vi "UpdatePump.vi"(8 "error in (no error)":errorcluster, 9 "DI":refnum<class "Sig_DI_Simple.lvclass">, 10 "DO in":refnum<class "Sig_DO_Simple.lvclass">, 11 "Pump_1AI_1DO_2DI in":refnum<class "Engine_1DI_2DO.lvclass">) -> (0 "error out":errorcluster, 2 "DO out":refnum<class "Sig_DO_Simple.lvclass">, 3 "Pump_1AI_1DO_2DI out":refnum<class "Engine_1DI_2DO.lvclass">)   [LabVIEW 2019, in "Engine_1DI_2DO.lvclass"]
uses:
  Engine_1DI_2DO.lvclass
  Sig_DI_Simple_class/Sig_DI_Simple.lvclass
  Sig_DO_Simple_class/Sig_DO_Simple.lvclass
  D:/H4000/src/Proccess_class/Proccess.lvclass
  Engine_1DI_2DO.lvclass/Engine_1DI_2DO.ctl
  Sig_DI_Simple_class/Sig_DI_Simple.lvclass/Sig_DI_Simple.ctl
  Sig_DA_class/Sig_DA.lvclass/Sig_DA.ctl
  Proccess_class/Proccess.lvclass/Proccess.ctl
  Sig_DO_Simple_class/Sig_DO_Simple.lvclass/Sig_DO_Simple.ctl
  TypeDef/StatePump.ctl
  Sig_DO_Simple_class/private/write_do_to_db.vi
  subvis/bool_change.vi
  Sig_DA_class/private/write_to_db.vi
  Proccess_class/Read TagName.vi
  Proccess_class/Read Logger.vi
  Sig_DA_class/Sig_DA.lvclass
  Logger_class/WriteEvent.vi
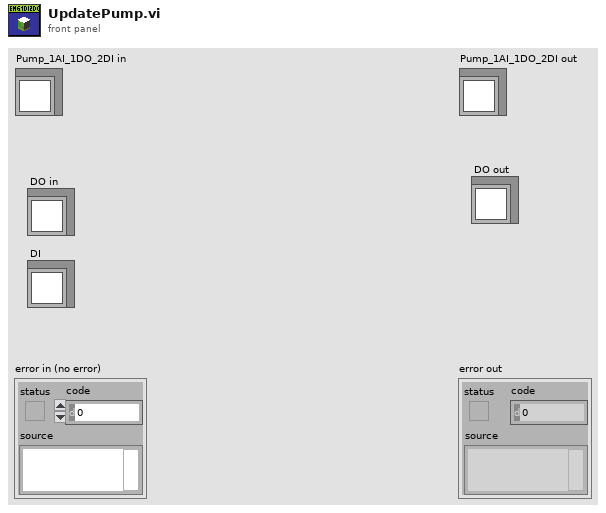
[diagram p1: front panel]
types:
  T1 = typedef "StatePump.ctl" = enum16{"Off", "TupningOn", "On", "TurningOff"}
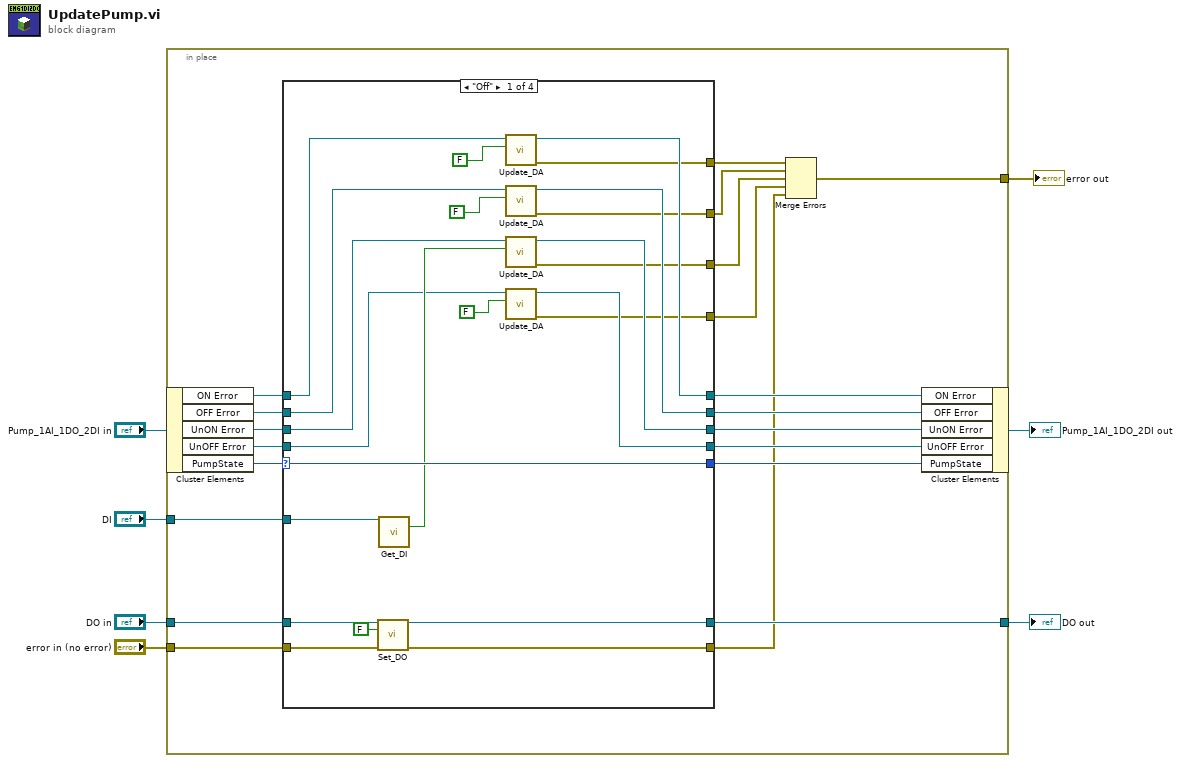
[diagram p0: block diagram]
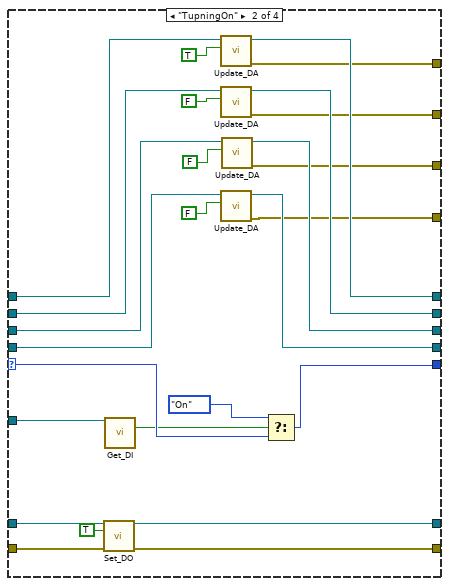
[diagram p2: hidden frame]
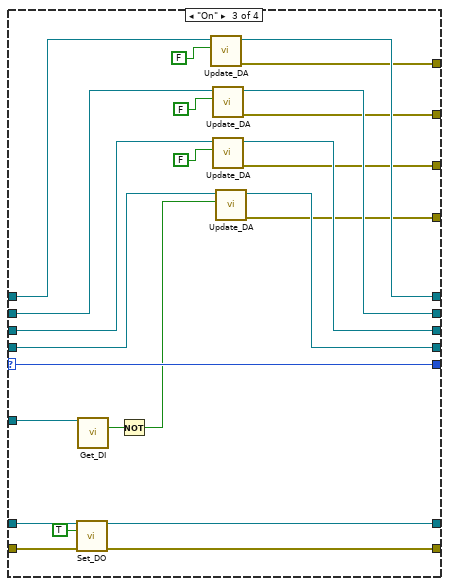
[diagram p3: hidden frame]
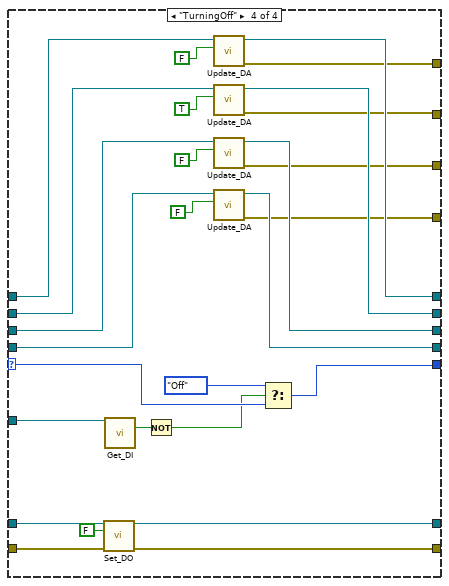
[diagram p4: hidden frame]
diagram:
  n1 = in-place {
    in-place-border: "DI" -> [w26]
    in-place-border: "DO in" -> [w24]
    in-place-border: [w23] -> w1
    in-place-border: "error in (no error)" -> [w22]
    in-place-border: [w8] -> w6
    n2 = in-place-cluster #1("Pump_1AI_1DO_2DI in") -> ("ON Error"=w19:refnum<class "Sig_DA.lvclass">, "OFF Error"=w17:refnum<class "Sig_DA.lvclass">, "UnON Error"=w21:refnum<class "Sig_DA.lvclass">, "UnOFF Error"=w15:refnum<class "Sig_DA.lvclass">, "PumpState"=w27:T1)
    n3 = case shown="\"Off\"" w27 {
      selector: w27 -> [w49 w75 w94 w126]
      tunnel: w26 -> [w50 w76 w100 w127]
      tunnel: [w49 w72 w94 w123] -> w25
      tunnel: w24 -> [w48 w71 w99 w122]
      tunnel: [w47 w70 w98 w121] -> w23
      tunnel: w22 -> [w45 w68 w96 w119]
      tunnel: [w44 w67 w95 w118] -> w9
      tunnel: w21 -> [w43 w58 w86 w108]
      tunnel: [w38 w65 w91 w114] -> w20
      tunnel: w19 -> [w39 w66 w92 w115]
      tunnel: [w35 w59 w87 w111] -> w18
      tunnel: w17 -> [w36 w60 w88 w112]
      tunnel: [w32 w55 w83 w106] -> w16
      tunnel: w15 -> [w33 w56 w84 w107]
      tunnel: [w42 w57 w85 w105] -> w14
      tunnel: [w31 w51 w77 w101] -> w10
      tunnel: [w30 w52 w78 w102] -> w11
      tunnel: [w29 w53 w79 w104] -> w12
      tunnel: [w28 w54 w80 w103] -> w13
      frame "Off" {
        n4 = call "Set_DO.vi"("reference in"=w48, "DO"=FALSE, "error in (no error)"=w45) -> ("reference out"=w47:refnum<class "Sig_DO_Simple.lvclass">, "error out"=w44:errorcluster)  [unwired: 11 in]
        n5 = call "Get_DI.vi"("reference in"=w50) -> ("DI"=w41:bool)  [unwired: 14 in]
        n6 = call "Update_DA.vi"("RAW"=FALSE, "Sig_DA in"=w39) -> ("error out"=w28:errorcluster, "Sig_DA out"=w38:refnum<class "Sig_DA.lvclass">)  [unwired: 7 in, 1 out]
        n7 = call "Update_DA.vi"("RAW"=FALSE, "Sig_DA in"=w36) -> ("error out"=w29:errorcluster, "Sig_DA out"=w35:refnum<class "Sig_DA.lvclass">)  [unwired: 7 in, 1 out]
        n8 = call "Update_DA.vi"("RAW"=w41, "Sig_DA in"=w43) -> ("error out"=w30:errorcluster, "Sig_DA out"=w42:refnum<class "Sig_DA.lvclass">)  [unwired: 7 in, 1 out]
        n9 = call "Update_DA.vi"("RAW"=FALSE, "Sig_DA in"=w33) -> ("error out"=w31:errorcluster, "Sig_DA out"=w32:refnum<class "Sig_DA.lvclass">)  [unwired: 7 in, 1 out]
      }
      frame "TupningOn" {
        n10 = call "Set_DO.vi"("reference in"=w71, "DO"=TRUE, "error in (no error)"=w68) -> ("reference out"=w70:refnum<class "Sig_DO_Simple.lvclass">, "error out"=w67:errorcluster)  [unwired: 11 in]
        n11 = call "Get_DI.vi"("reference in"=w76) -> ("DI"=w74:bool)  [unwired: 14 in]
        n12 = call "Update_DA.vi"("RAW"=TRUE, "Sig_DA in"=w66) -> ("error out"=w54:errorcluster, "Sig_DA out"=w65:refnum<class "Sig_DA.lvclass">)  [unwired: 7 in, 1 out]
        n13 = call "Update_DA.vi"("RAW"=FALSE, "Sig_DA in"=w60) -> ("error out"=w53:errorcluster, "Sig_DA out"=w59:refnum<class "Sig_DA.lvclass">)  [unwired: 7 in, 1 out]
        n14 = call "Update_DA.vi"("RAW"=FALSE, "Sig_DA in"=w56) -> ("error out"=w51:errorcluster, "Sig_DA out"=w55:refnum<class "Sig_DA.lvclass">)  [unwired: 7 in, 1 out]
        n15 = call "Update_DA.vi"("RAW"=FALSE, "Sig_DA in"=w58) -> ("error out"=w52:errorcluster, "Sig_DA out"=w57:refnum<class "Sig_DA.lvclass">)  [unwired: 7 in, 1 out]
        n16 = Select(t=StatePump."On", s=w74, f=w75) -> (s? t:f=w72:T1)
      }
      frame "On" {
        n17 = call "Set_DO.vi"("reference in"=w99, "DO"=TRUE, "error in (no error)"=w96) -> ("reference out"=w98:refnum<class "Sig_DO_Simple.lvclass">, "error out"=w95:errorcluster)  [unwired: 11 in]
        n18 = call "Get_DI.vi"("reference in"=w100) -> ("DI"=w82:bool)  [unwired: 14 in]
        n19 = Not(x=w82) -> (.not. x?=w81:bool)
        n20 = call "Update_DA.vi"("RAW"=FALSE, "Sig_DA in"=w92) -> ("error out"=w80:errorcluster, "Sig_DA out"=w91:refnum<class "Sig_DA.lvclass">)  [unwired: 7 in, 1 out]
        n21 = call "Update_DA.vi"("RAW"=FALSE, "Sig_DA in"=w88) -> ("error out"=w79:errorcluster, "Sig_DA out"=w87:refnum<class "Sig_DA.lvclass">)  [unwired: 7 in, 1 out]
        n22 = call "Update_DA.vi"("RAW"=FALSE, "Sig_DA in"=w86) -> ("error out"=w78:errorcluster, "Sig_DA out"=w85:refnum<class "Sig_DA.lvclass">)  [unwired: 7 in, 1 out]
        n23 = call "Update_DA.vi"("RAW"=w81, "Sig_DA in"=w84) -> ("error out"=w77:errorcluster, "Sig_DA out"=w83:refnum<class "Sig_DA.lvclass">)  [unwired: 7 in, 1 out]
      }
      frame "TurningOff" {
        n24 = call "Set_DO.vi"("reference in"=w122, "DO"=FALSE, "error in (no error)"=w119) -> ("reference out"=w121:refnum<class "Sig_DO_Simple.lvclass">, "error out"=w118:errorcluster)  [unwired: 11 in]
        n25 = call "Get_DI.vi"("reference in"=w127) -> ("DI"=w125:bool)  [unwired: 14 in]
        n26 = Not(x=w125) -> (.not. x?=w117:bool)
        n27 = call "Update_DA.vi"("RAW"=FALSE, "Sig_DA in"=w115) -> ("error out"=w103:errorcluster, "Sig_DA out"=w114:refnum<class "Sig_DA.lvclass">)  [unwired: 7 in, 1 out]
        n28 = call "Update_DA.vi"("RAW"=TRUE, "Sig_DA in"=w112) -> ("error out"=w104:errorcluster, "Sig_DA out"=w111:refnum<class "Sig_DA.lvclass">)  [unwired: 7 in, 1 out]
        n29 = call "Update_DA.vi"("RAW"=FALSE, "Sig_DA in"=w108) -> ("error out"=w102:errorcluster, "Sig_DA out"=w105:refnum<class "Sig_DA.lvclass">)  [unwired: 7 in, 1 out]
        n30 = call "Update_DA.vi"("RAW"=FALSE, "Sig_DA in"=w107) -> ("error out"=w101:errorcluster, "Sig_DA out"=w106:refnum<class "Sig_DA.lvclass">)  [unwired: 7 in, 1 out]
        n31 = Select(t=StatePump."Off", s=w117, f=w126) -> (s? t:f=w123:T1)
      }
    }
    n32 = Merge Errors(w13, w12, w11, w10, w9) -> (w8:errorcluster)
    n33 = in-place-cluster #1("ON Error"=w20, "OFF Error"=w18, "UnON Error"=w14, "UnOFF Error"=w16, "PumpState"=w25) -> (→"Pump_1AI_1DO_2DI out":refnum<class "Engine_1DI_2DO.lvclass">)
  }
  "error out" <- w6
  "DO out" <- w1
